vi "TargetsMingledotcom.vi"(10 "Left Targets":T1[](array[typedef]), 11 "Right Targets":T1[](array[typedef])) -> (3 "Target Set":T2(array[cluster]))   [LabVIEW 2014]
uses:
  target type.ctl
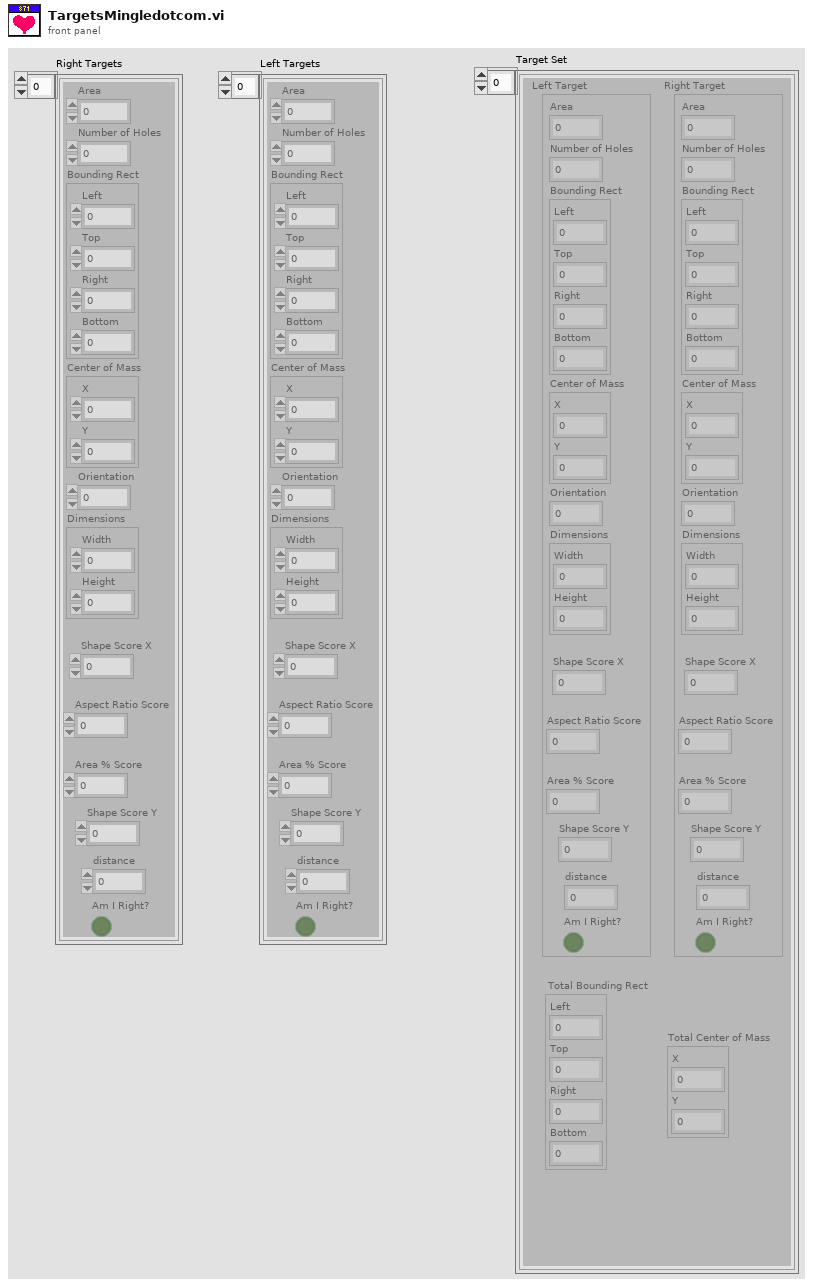
[diagram p1: front panel]
types:
  T1 = typedef "target type.ctl" = cluster{"Area":dbl, "Number of Holes":dbl, "Bounding Rect":cluster{"Left":dbl, "Top":dbl, "Right":dbl, "Bottom":dbl}, "Center of Mass":cluster{"X":dbl, "Y":dbl}, "Orientation":dbl, "Dimensions":cluster{"Width":dbl, "Height":dbl}, "Shape Score X":dbl, "Aspect Ratio Score":dbl, "Area % Score":dbl, "Shape Score Y":dbl, "Am I Right?":bool, "distance":dbl}
  T2 = cluster{"Left Target":T1, "Right Target":T1, "Total Bounding Rect":cluster{"Left":dbl, "Top":dbl, "Right":dbl, "Bottom":dbl}, "Total Center of Mass":cluster{"X":dbl, "Y":dbl}}[]
  T3 = cluster{"Left Target":T1, "Right Target":T1, "Total Bounding Rect":cluster{"Left":dbl, "Top":dbl, "Right":dbl, "Bottom":dbl}, "Total Center of Mass":cluster{"X":dbl, "Y":dbl}}
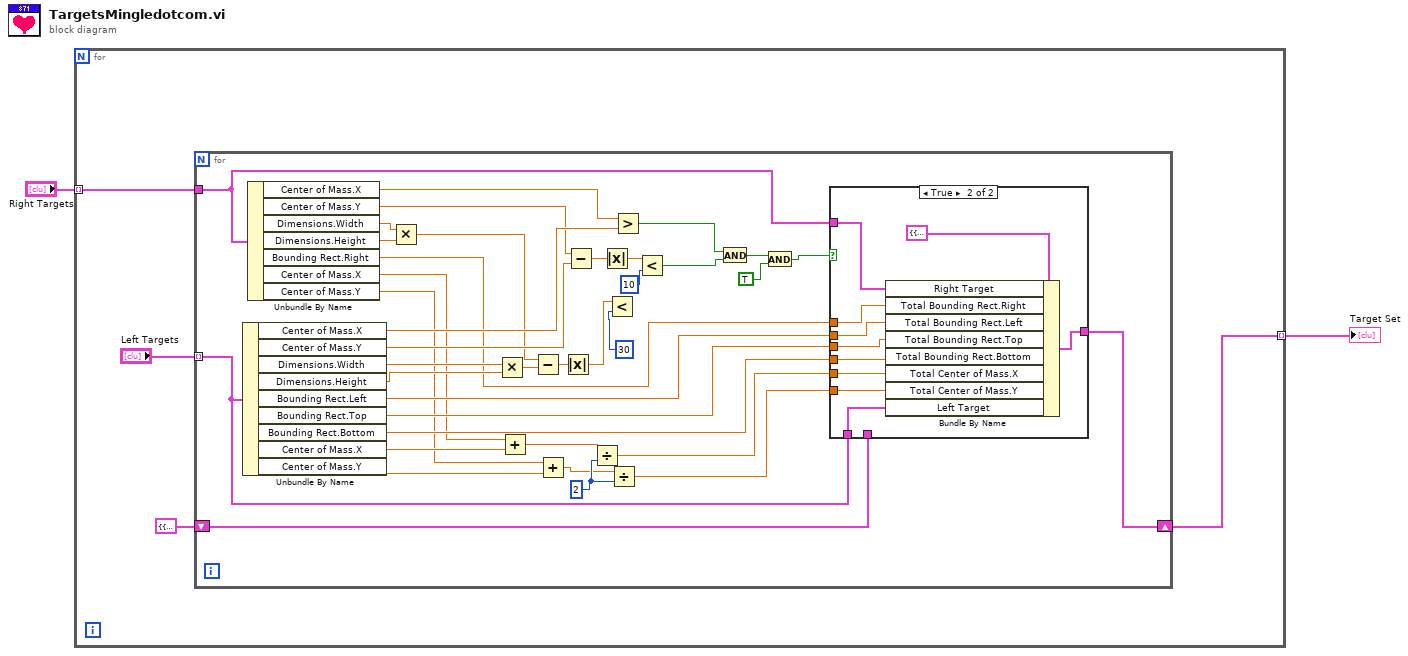
[diagram p0: block diagram]
diagram:
  n1 = for {
    tunnel: "Right Targets" -> [w6] mode=indexing
    tunnel: [w4] -> w1 mode=indexing
    n2 = for {
      tunnel: w6 -> [w28]
      tunnel: "Left Targets" -> [w27] mode=indexing
      shift-right: [w22] -> w4
      shift-left: T3 {"Left Target"={"Area"=0.0, "Number of Holes"=0.0, "Bounding Rect"={"Left"=0.0, "Top"=0.0, "Right"=0.0, "Bottom"=0.0}, "Center of Mass"={"X"=0.0, "Y"=0.0}, "Orientation"=0.0, "Dimensions"={"Width"=0.0, "Height"=0.0}, "Shape Score X"=0.0, "Aspect Ratio Score"=0.0, "Area % Score"=0.0, "Shape Score Y"=0.0, "Am I Right?"=FALSE, "distance"=0.0}, "Right Target"={"Area"=0.0, "Number of Holes"=0.0, "Bounding Rect"={"Left"=0.0, "Top"=0.0, "Right"=0.0, "Bottom"=0.0}, "Center of Mass"={"X"=0.0, "Y"=0.0}, "Orientation"=0.0, "Dimensions"={"Width"=0.0, "Height"=0.0}, "Shape Score X"=0.0, "Aspect Ratio Score"=0.0, "Area % Score"=0.0, "Shape Score Y"=0.0, "Am I Right?"=FALSE, "distance"=0.0}, "Total Bounding Rect"={"Left"=0.0, "Top"=0.0, "Right"=0.0, "Bottom"=0.0}, "Total Center of Mass"={"X"=0.0, "Y"=0.0}} ("Cluster") -> [w21]
      w15 = 2
      n3 = Unbundle By Name(w27) -> ("Center of Mass.X"=w43:dbl, "Center of Mass.Y"=w40:dbl, "Dimensions.Width"=w35:dbl, "Dimensions.Height"=w34:dbl, "Bounding Rect.Left"=w25:dbl, "Bounding Rect.Top"=w24:dbl, "Bounding Rect.Bottom"=w23:dbl, "Center of Mass.X"=w11:dbl, "Center of Mass.Y"=w10:dbl)
      n4 = Unbundle By Name(w28) -> ("Center of Mass.X"=w44:dbl, "Center of Mass.Y"=w41:dbl, "Dimensions.Width"=w37:dbl, "Dimensions.Height"=w36:dbl, "Bounding Rect.Right"=w26:dbl, "Center of Mass.X"=w12:dbl, "Center of Mass.Y"=w9:dbl)
      n5 = Multiply(x=w37, y=w36) -> (x*y=w32:dbl)
      n6 = Multiply(x=w35, y=w34) -> (x*y=w33:dbl)
      n7 = Add(x=w12, y=w11) -> (x+y=w13:dbl)
      n8 = Subtract(x=w32, y=w33) -> (x-y=w31:dbl)
      n9 = Add(x=w9, y=w10) -> (x+y=w14:dbl)
      n10 = Absolute Value(x=w31) -> (abs(x)=w20:dbl)
      n11 = Subtract(x=w41, y=w40) -> (x-y=w42:dbl)
      n12 = Divide(x=w13, y=w15) -> (x/y=w8:dbl)
      n13 = Absolute Value(x=w42) -> (abs(x)=w18:dbl)
      n14 = Less?(x=w20, y=30) -> ()  [unwired: 1 out]
      n15 = Divide(x=w14, y=w15) -> (x/y=w7:dbl)
      n16 = Greater?(x=w44, y=w43) -> (0:w39:bool)
      n17 = Less?(x=w18, y=10) -> (x < y?=w38:bool)
      n18 = And(x=w39, y=w38) -> (x .and. y?=w30:bool)
      n19 = And(x=w30, y=TRUE) -> (x .and. y?=w29:bool)
      n20 = case shown="True" w29 {
        tunnel: w28 -> [_ w51]
        tunnel: w27 -> [_ w48]
        tunnel: [w45 w50] -> w22
        tunnel: w26 -> [_ w55]
        tunnel: w25 -> [_ w54]
        tunnel: w24 -> [_ w53]
        tunnel: w23 -> [_ w52]
        tunnel: w21 -> [w45 _]
        tunnel: w8 -> [_ w47]
        tunnel: w7 -> [_ w46]
        frame False {
        }
        frame True {
          n21 = Bundle By Name(cluster=T3 {"Left Target"={"Area"=0.0, "Number of Holes"=0.0, "Bounding Rect"={"Left"=0.0, "Top"=0.0, "Right"=0.0, "Bottom"=0.0}, "Center of Mass"={"X"=0.0, "Y"=0.0}, "Orientation"=0.0, "Dimensions"={"Width"=0.0, "Height"=0.0}, "Shape Score X"=0.0, "Aspect Ratio Score"=0.0, "Area % Score"=0.0, "Shape Score Y"=0.0, "Am I Right?"=FALSE, "distance"=0.0}, "Right Target"={"Area"=0.0, "Number of Holes"=0.0, "Bounding Rect"={"Left"=0.0, "Top"=0.0, "Right"=0.0, "Bottom"=0.0}, "Center of Mass"={"X"=0.0, "Y"=0.0}, "Orientation"=0.0, "Dimensions"={"Width"=0.0, "Height"=0.0}, "Shape Score X"=0.0, "Aspect Ratio Score"=0.0, "Area % Score"=0.0, "Shape Score Y"=0.0, "Am I Right?"=FALSE, "distance"=0.0}, "Total Bounding Rect"={"Left"=0.0, "Top"=0.0, "Right"=0.0, "Bottom"=0.0}, "Total Center of Mass"={"X"=0.0, "Y"=0.0}} ("Cluster"), "Right Target"=w51, "Total Bounding Rect.Right"=w55, "Total Bounding Rect.Left"=w54, "Total Bounding Rect.Top"=w53, "Total Bounding Rect.Bottom"=w52, "Total Center of Mass.X"=w47, "Total Center of Mass.Y"=w46, "Left Target"=w48) -> (w50:T3)
        }
      }
    }
  }
  "Target Set" <- w1
